vi "ProtocolControl2.vi"() -> ()   [LabVIEW 2016]
uses:
  ProtocolStatus.ctl
  <vilib>/xml/Close Reference(Node).vi
  <vilib>/xml/Load XML File.vi
  <vilib>/xml/NI_XML.lvlib
  <resource>/objmgr/DOMUserDefRef.rc
panel:
  out "Time to Next":dbl format="%#.2f"
  out "Time to Next Subsession":dbl caption="Time to Next"
  out "Current Subsession":string caption="Name"
  out "Time of Current Subsession":dbl caption="Time"
  out "Current Subsession Idx":i32 caption="Index"
  in  "Engage":bool
  in  "Subject ID":string
  out "Pause Time":dbl format="%#.2f"
  out "Record Time":dbl format="%#.2f"
  out "Session Time (s)":dbl
  out "Current Session":dbl(slide) min=0.0 max=600.0 scale=0.0..180.0
  out "Current Time":dbl format="%#.2f"
  out "File Name":string
  out "Suggestions":string
  in  "Close Protocol":bool
  in  "Pause Session":bool
  in  "Start Session":bool
  in  "Load Protocol":bool
  in  "Sessions":i32(listbox)
  in  "XML File Path":path
  # "Current Subsession"
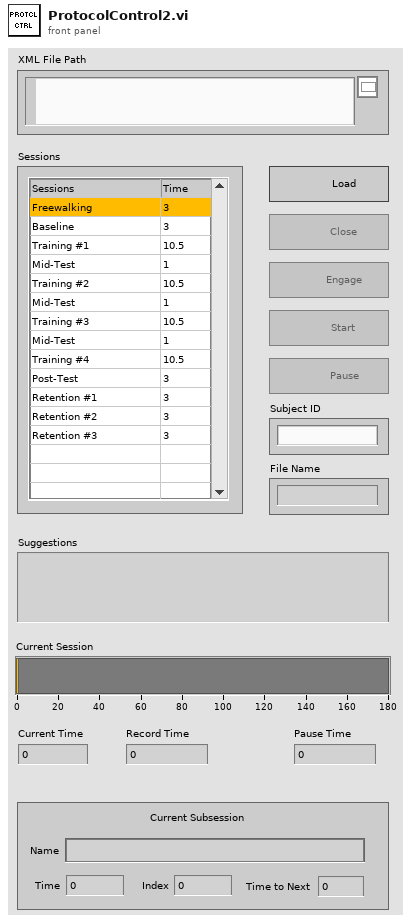
[diagram p1: front panel]
types:
  T1 = typedef "ProtocolStatus.ctl" = enum16{"No Protocol", "Protocol Idle", "Protocol Start", "Protocol Pause"}
  T2 = enum8{"Enabled", "Disabled", "Disabled and Grayed Out"}
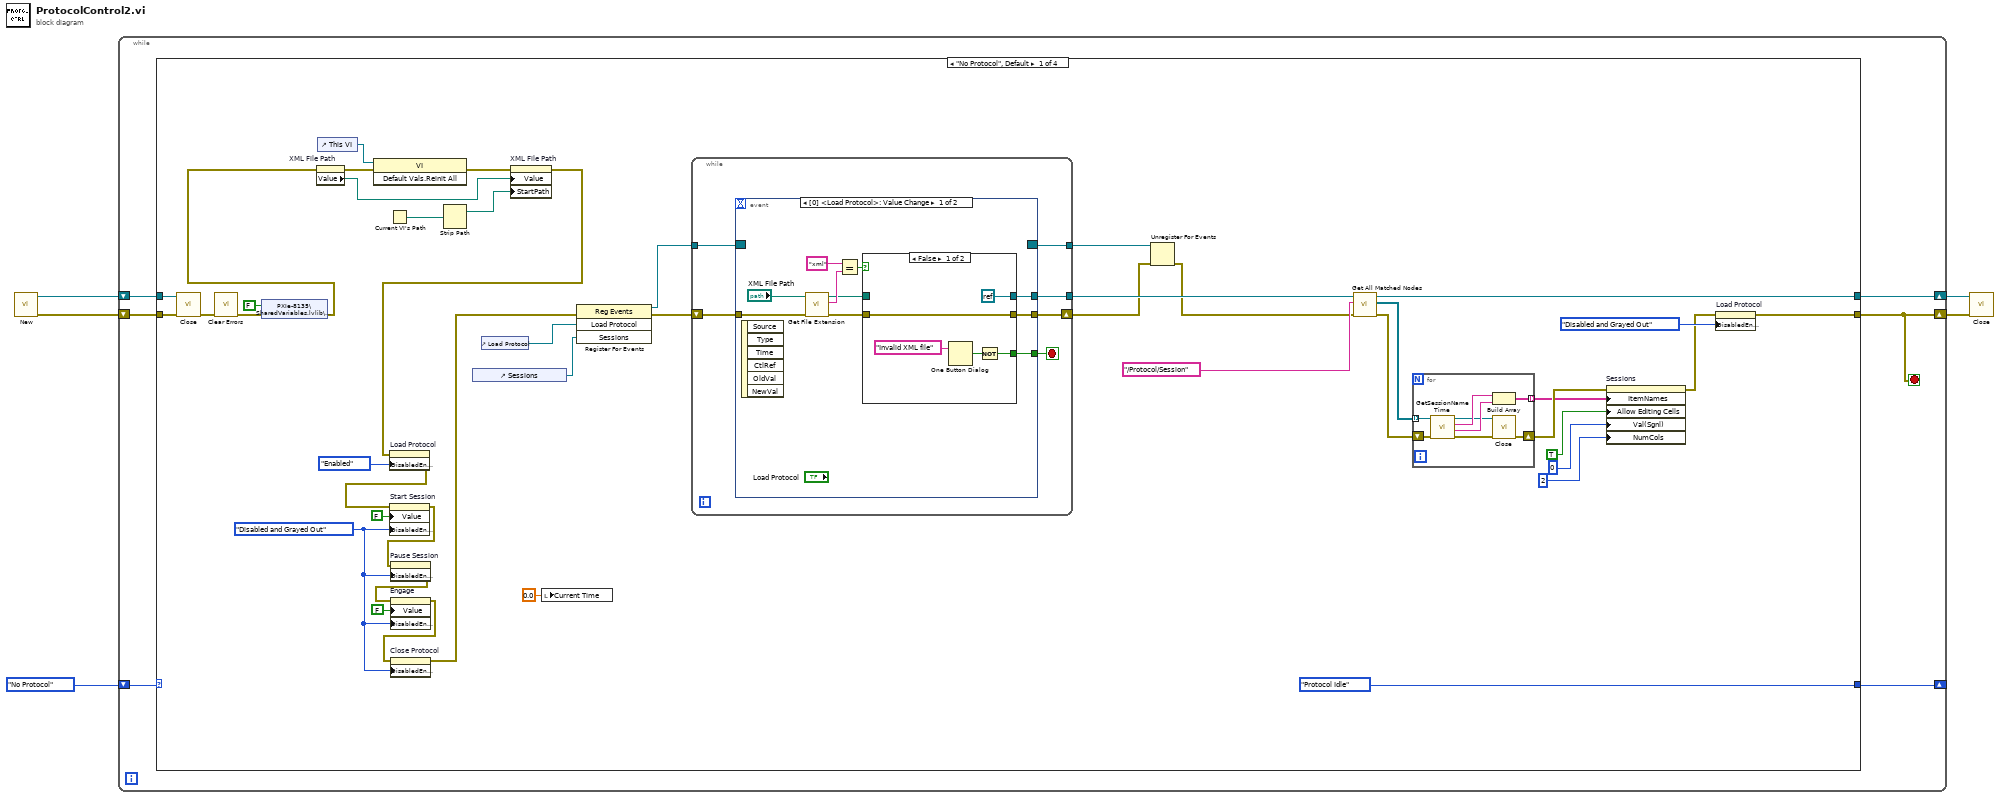
[diagram p0: block diagram]
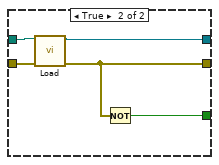
[diagram p2: hidden frame]
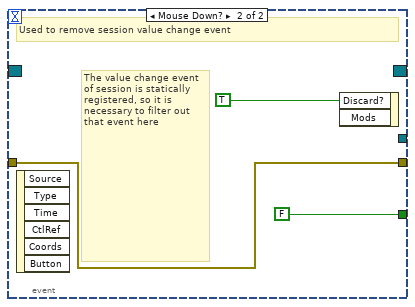
[diagram p3: hidden frame]
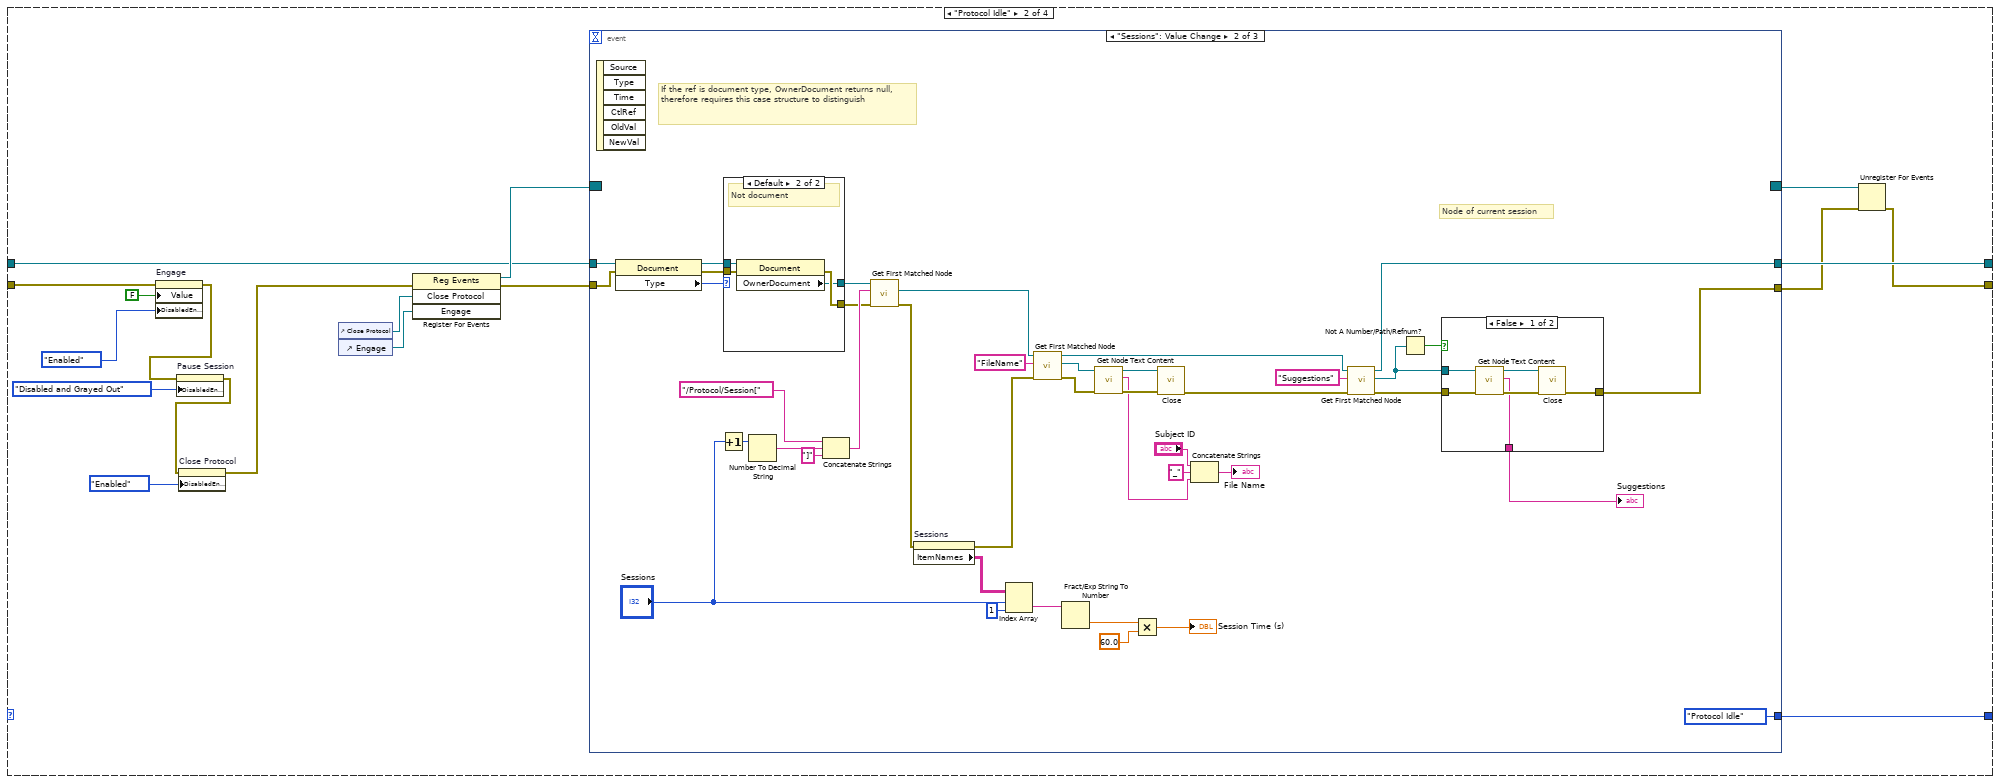
[diagram p4: hidden frame]
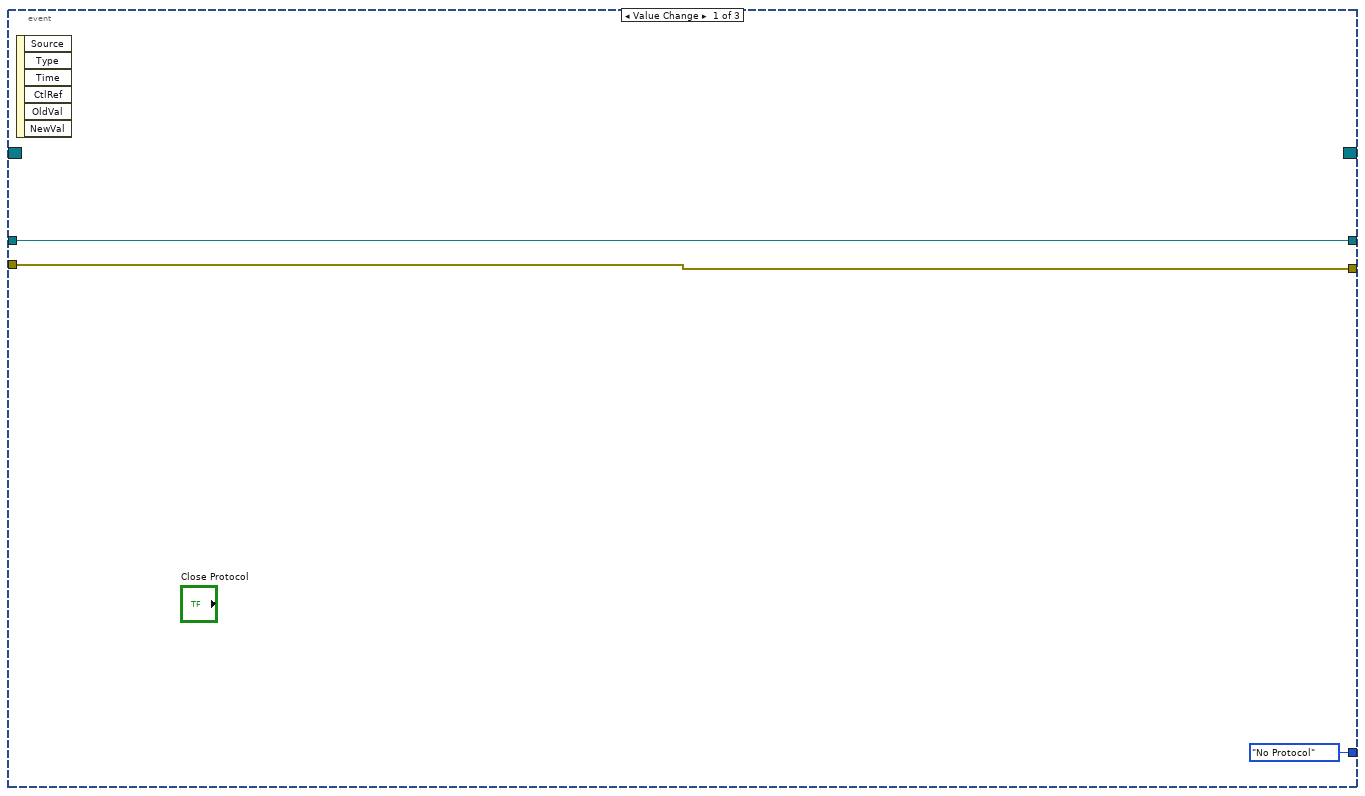
[diagram p5: hidden frame]
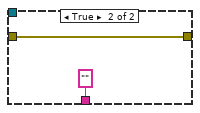
[diagram p7: hidden frame]
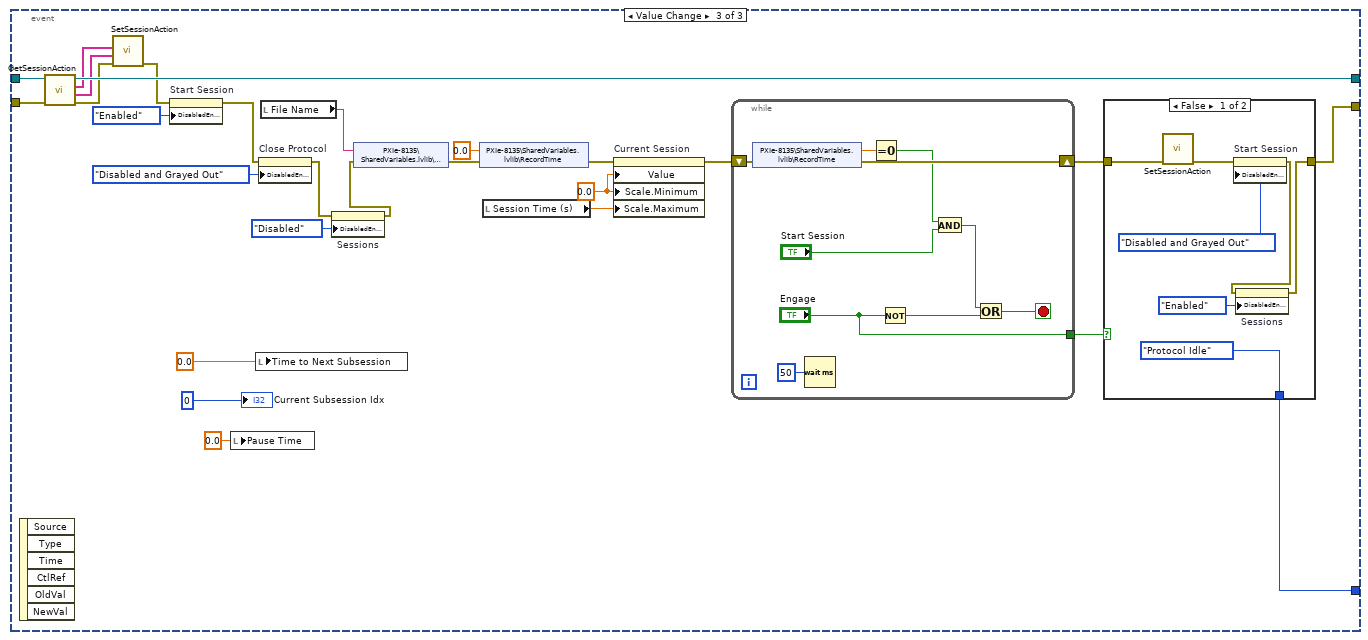
[diagram p8: hidden frame]
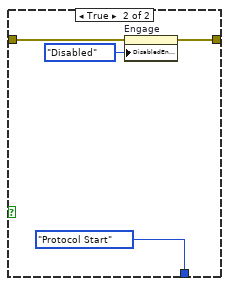
[diagram p9: hidden frame]
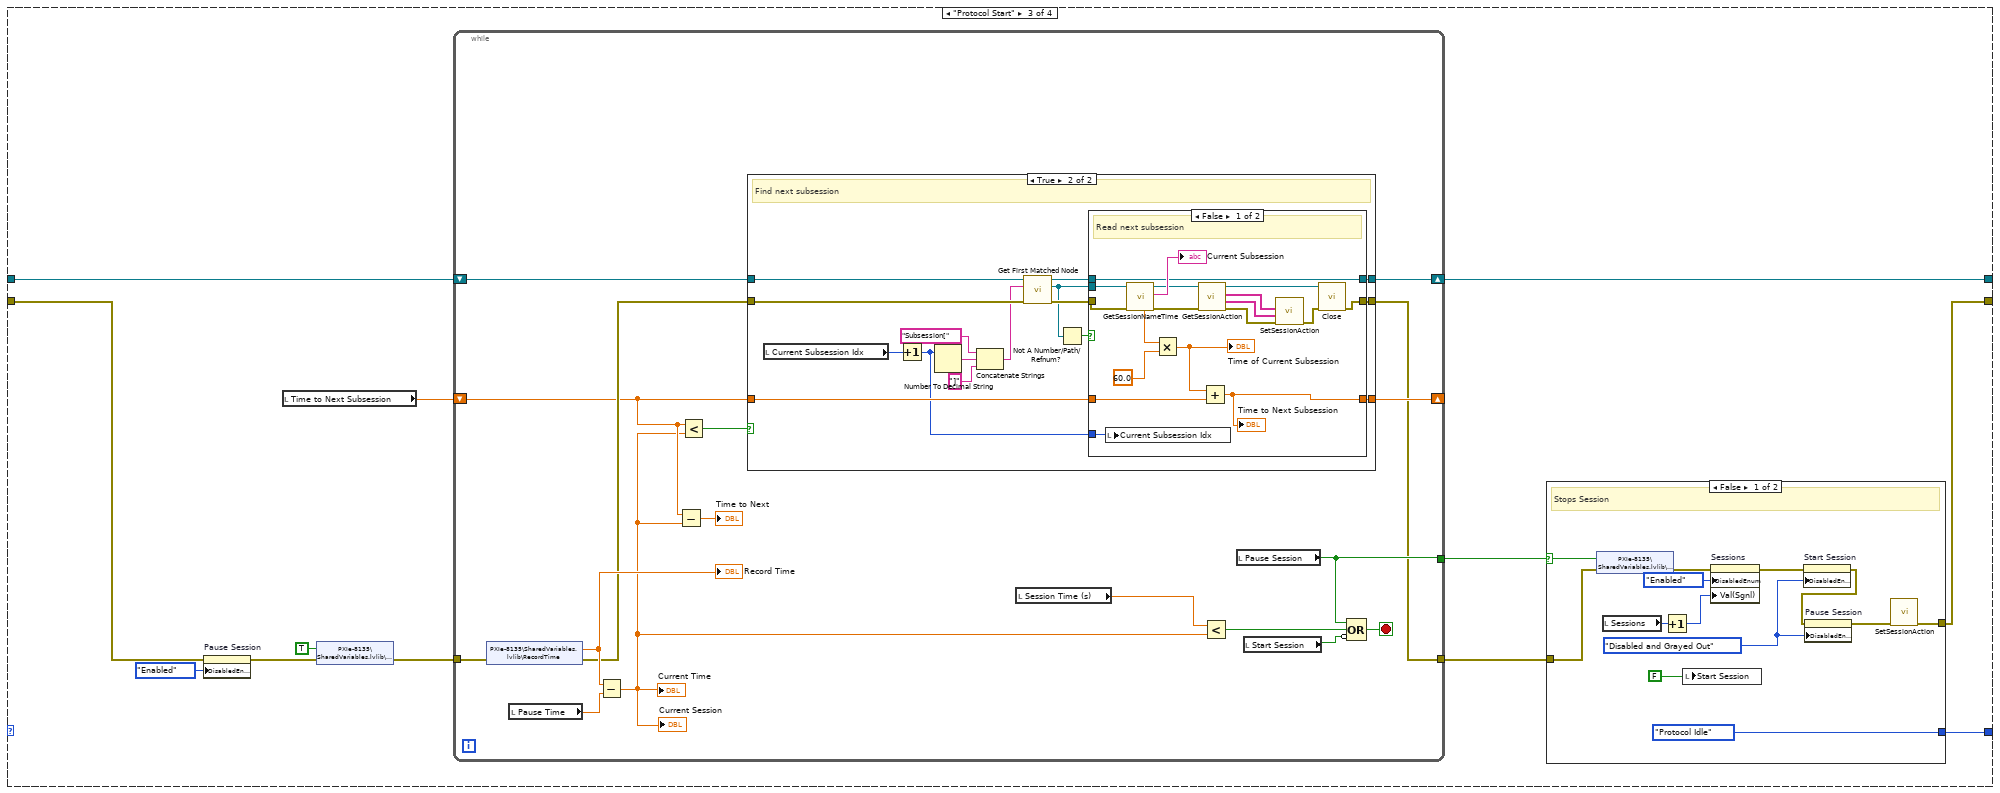
[diagram p10: hidden frame]
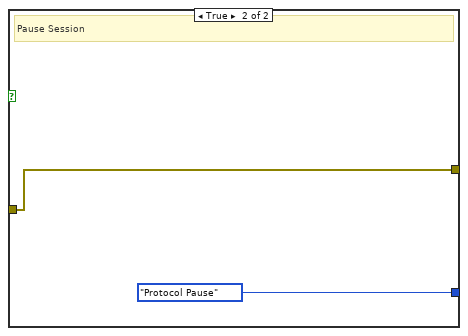
[diagram p11: hidden frame]
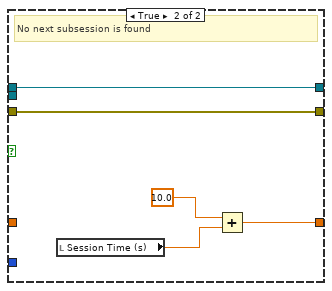
[diagram p13: hidden frame]
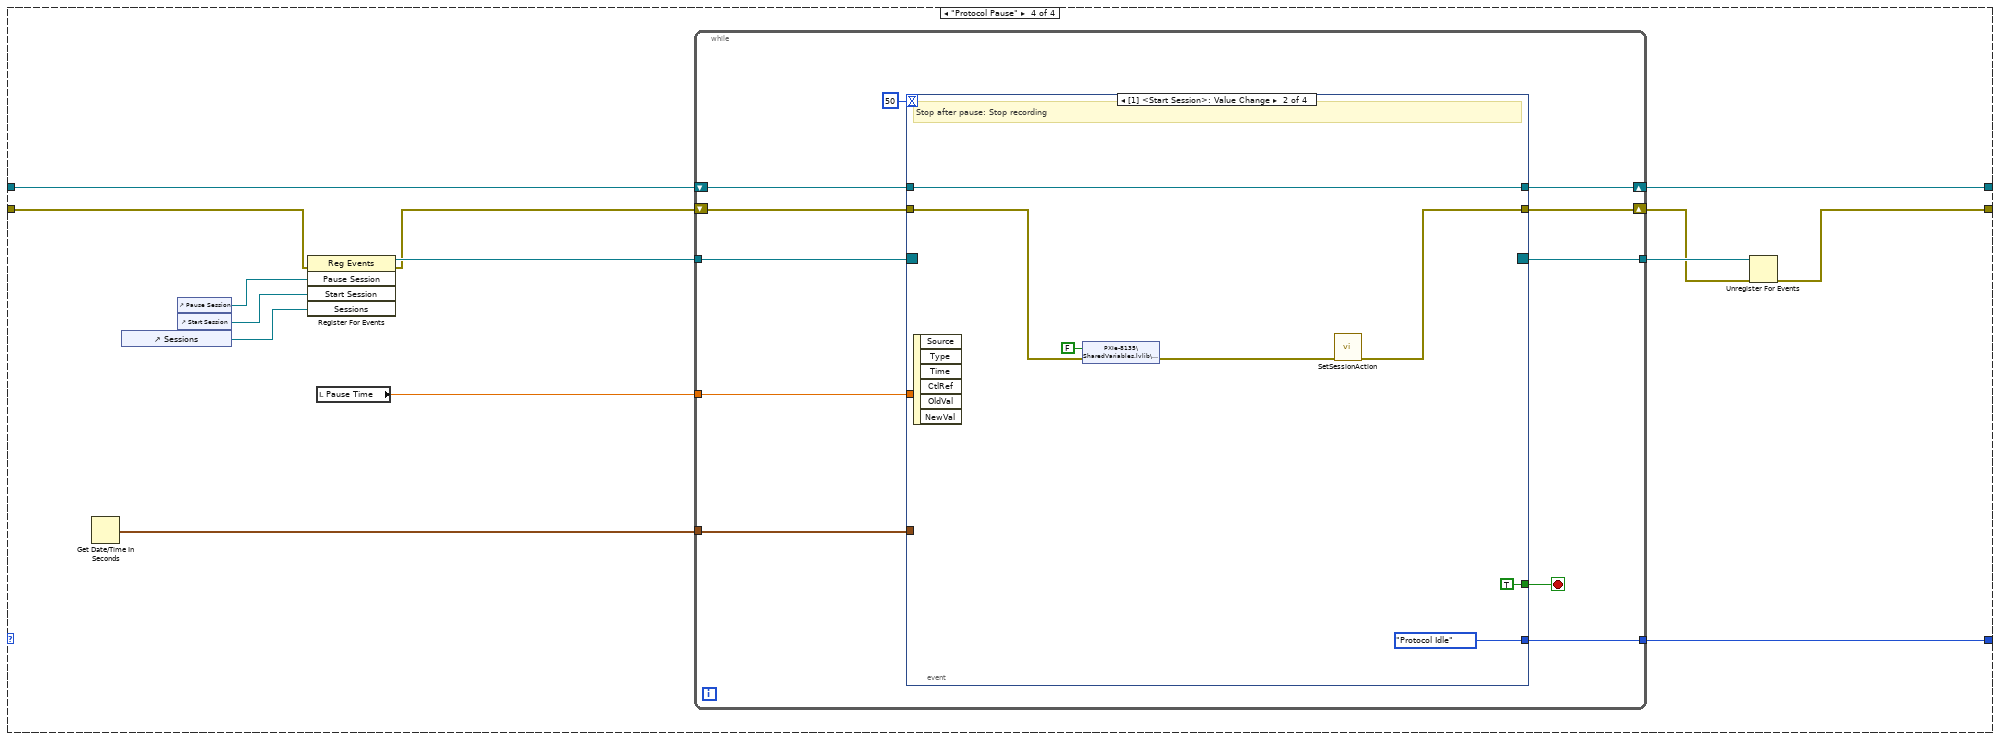
[diagram p14: hidden frame]
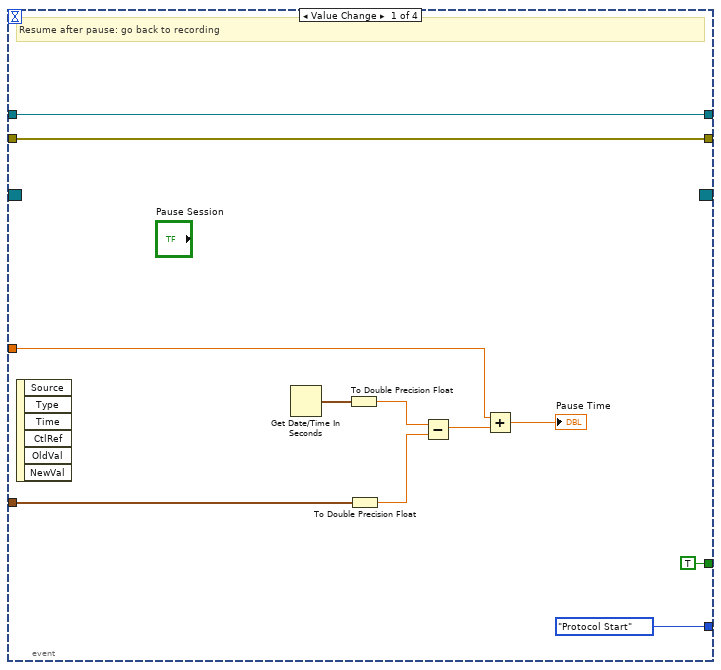
[diagram p15: hidden frame]
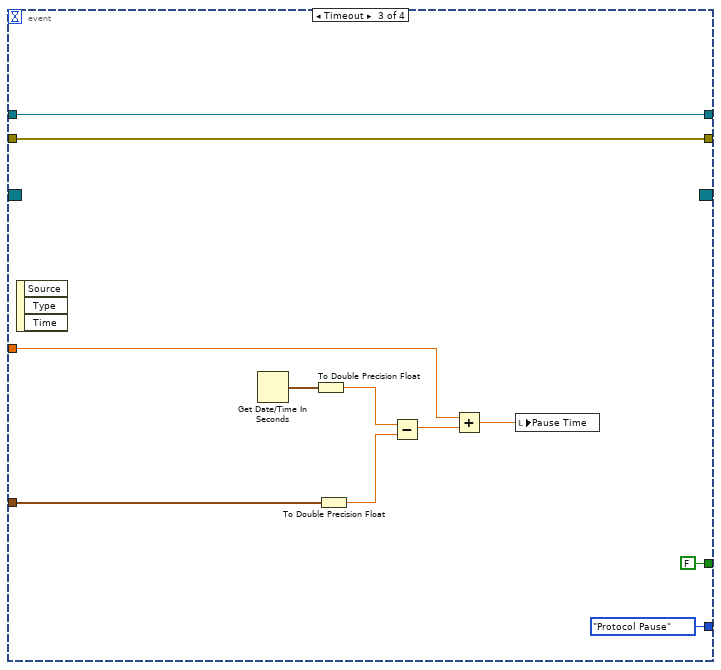
[diagram p16: hidden frame]
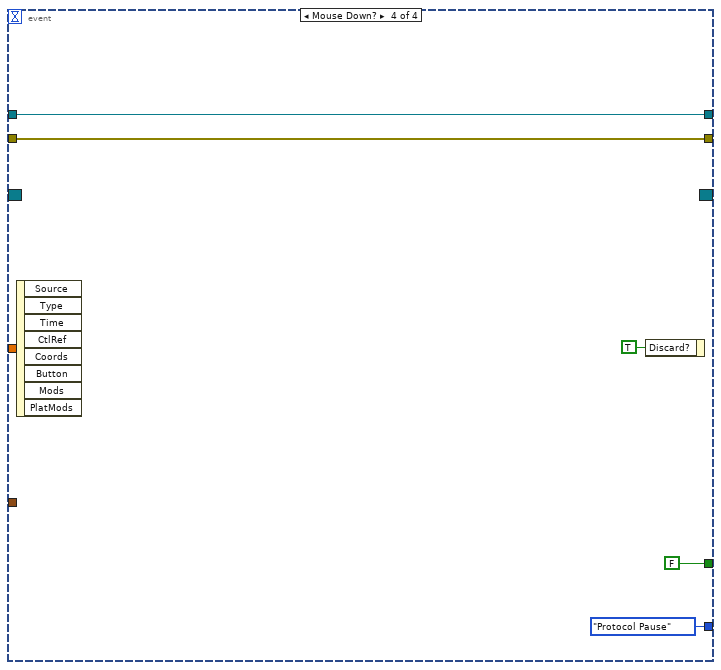
[diagram p17: hidden frame]
diagram:
  n1 = call <vilib>:"New.vi"() -> ("error out"=w3:errorcluster, "DOM document out"=w4:refnum<k20>)  [unwired: 8 in]
  n2 = while {
    shift-right: [w10] -> w2
    shift-left: w4 -> [w9]
    shift-right: [w6] -> w1
    shift-left: w3 -> [w8]
    shift-right: [w7] -> _
    shift-left: ProtocolStatus."No Protocol" -> [w11]
    stop <- w6 stop-if-true
    n3 = case shown="\"No Protocol\", Default" w11 {
      tunnel: [w48 w109 w226 w314] -> w10
      tunnel: w9 -> [w55 w104 w219 w315]
      tunnel: w8 -> [w54 w102 w218 w308]
      tunnel: [w24 w94 w223 w304] -> w6
      tunnel: [ProtocolStatus."Protocol Idle" w110 w222 w316] -> w7
      frame "No Protocol", Default {
        w25 = T2."Disabled and Grayed Out" ("Disabled")
        n4 = call-poly <vilib>:"Close.vi"("error in (no error)"=w54, "node"=w55) -> ("error out"=w21:errorcluster)  [unwired: 7 in]
        n5 = call <vilib>:"Clear Errors.vi"("error in (no error)"=w21) -> ("error out"=w20:errorcluster)  [unwired: 5 in, 1 out]
        n6 = shared-variable "PXIe-8135\\SharedVariables.lvlib\\Record?"(FALSE ("Record?"), error in=w20) -> (error out=w18:errorcluster)
        n7 = property on="XML File Path" class="Path"(error in=w18) -> (error out=w14:errorcluster, "Value"=w13:path)  [unwired: 1 in, 1 out]
        n8 = control-ref of="This VI"() -> (w16:refnum<vi>)
        n9 = invoke class="VI" method="Default Vals.Reinit All"(reference=w16, error in=w14) -> (error out=w15:errorcluster)  [unwired: 1 in, 2 out]
        n10 = Current VI's Path() -> (path=w17:path)
        n11 = Strip Path(path=w17) -> (stripped path=w12:path)  [unwired: 1 out]
        n12 = control-ref of="Sessions"() -> (w36:refnum<vi>)
        n13 = control-ref of="Load Protocol"() -> (w35:refnum<vi>)
        n14 = property on="XML File Path" class="Path"(error in=w15, "Value"=w13, "StartPath"=w12) -> (error out=w19:errorcluster)  [unwired: 1 in, 1 out]
        n15 = property on="Load Protocol" class="Bool"(error in=w19, "DisabledEnum"=T2."Enabled" ("Disabled")) -> (error out=w37:errorcluster)  [unwired: 1 in, 1 out]
        n16 = property on="Start Session" class="Bool (strict)"(error in=w37, "Value"=FALSE ("Start Session"), "DisabledEnum"=w25) -> (error out=w29:errorcluster)  [unwired: 1 in, 1 out]
        n17 = property on="Pause Session" class="Bool (strict)"(error in=w29, "DisabledEnum"=w25) -> (error out=w28:errorcluster)  [unwired: 1 in, 1 out]
        n18 = property on="Engage" class="Bool (strict)"(error in=w28, "Value"=FALSE ("Engage"), "DisabledEnum"=w25) -> (error out=w27:errorcluster)  [unwired: 1 in, 1 out]
        n19 = property on="Close Protocol" class="Bool"(error in=w27, "DisabledEnum"=w25) -> (error out=w26:errorcluster)  [unwired: 1 in, 1 out]
        n20 = local write "Current Time"(0.0 ("Current Time")) -> ()
        n21 = register-events(error in=w26, w35, w36) -> (reference out=w33:refnum<event-registration>, error out=w34:errorcluster)  [unwired: 1 in]
        n22 = while {
          tunnel: [w61] -> w49
          shift-right: [w58] -> w31
          shift-left: w34 -> [w56]
          tunnel: w33 -> [w59]
          tunnel: [w57] -> w32
          stop <- w60 stop-if-true
          n23 = event shown="[0] <Load Protocol>: Value Change" {
            selector: w59 -> [_ _]
            dyn-events: [_ _] -> w57
            timeout: _ -> [_ _]
            tunnel: [w63 _] -> w61
            tunnel: w56 -> [w67 w82]
            tunnel: [w62 FALSE] -> w60
            tunnel: [w64 w82] -> w58
            event Value Change {
              n24 = event-data() -> ()  [unwired: 1 in, 6 out]
              n25 = call <vilib>:"Get File Extension.vi"("error in (no error)"=w67, "file"="XML File Path") -> ("error out"=w66:errorcluster, "lowercase file extension"=w68:string, "dup file"=w65:path)  [unwired: 5 in, 2 out]
              n26 = Equal?(x="xml" ("y"), y=w68) -> (x = y?=w71:bool)
              n27 = case shown="False" w71 {
                tunnel: w66 -> [w75 w80]
                tunnel: w65 -> [_ w81]
                tunnel: [w75 w78] -> w64
                tunnel: [refnum<k0> refnum w79] -> w63
                tunnel: [w73 w77] -> w62
                frame False {
                  n28 = One Button Dialog(message="Invalid XML file") -> (true=w74:bool)  [unwired: 1 in]
                  n29 = Not(x=w74) -> (.not. x?=w73:bool)
                }
                frame True {
                  n30 = call-poly <vilib>:"Load.vi"("path to XML document"=w81, "error in (no error)"=w80) -> ("DOM document out"=w79:refnum<k20>, "error out"=w78:errorcluster)  [unwired: 11 in, 1 out]
                  n31 = Not(x=w78) -> (.not. x?=w77:bool)
                }
              }
            }
            event Mouse Down? {
              # "The value change event of session is statically registered, so it is necessary to filter out that event here"
              # "Used to remove session value change event"
              n32 = event-data() -> ()  [unwired: 1 in, 6 out]
              n33 = event-data("Discard?"=TRUE) -> ()  [unwired: 2 in, 1 out]
            }
          }
        }
        n34 = Unregister For Events(event registration refnum=w32, error in=w31) -> (error out=w30:errorcluster)
        n35 = call <vilib>:"Get All Matched Nodes.vi"("error in (no error)"=w30, "XPath expression"="/Protocol/Session", "node in"=w49) -> ("error out"=w52:errorcluster, "node result array"=w50:refnum<k20>[], "node out"=w48:refnum<k20>)  [unwired: 6 in]
        n36 = for {
          tunnel: w50 -> [w85] mode=indexing
          shift-right: [w86] -> w47
          shift-left: w52 -> [w92]
          tunnel: [w89] -> w43 mode=indexing
          n37 = call "GetSessionNameTime.vi"("error in (no error)"=w92, "Refnum in"=w85) -> ("error out"=w88:errorcluster, "Session Time"=w91:string, "Session Name"=w90:string, "node out"=w87:refnum<k20>)  [unwired: 5 in, 1 out]
          n38 = Build Array(w90, w91) -> (w89:string[])
          n39 = call-poly <vilib>:"Close.vi"("error in (no error)"=w88, "node"=w87) -> ("error out"=w86:errorcluster)  [unwired: 7 in]
        }
        n40 = property on="Sessions" class="MCListbox (strict)"(error in=w47, "ItemNames"=w43, "Allow Editing Cells"=TRUE, "Val(Sgnl)"=0 ("Protocol"), "NumCols"=u32 2 ("Number of Columns")) -> (error out=w39:errorcluster)  [unwired: 1 in, 1 out]
        n41 = property on="Load Protocol" class="Bool"(error in=w39, "DisabledEnum"=T2."Disabled and Grayed Out" ("Disabled")) -> (error out=w24:errorcluster)  [unwired: 1 in, 1 out]
      }
      frame "Protocol Idle" {
        n42 = property on="Engage" class="Bool (strict)"(error in=w102, "Value"=FALSE ("Engage"), "DisabledEnum"=T2."Enabled" ("Disabled")) -> (error out=w99:errorcluster)  [unwired: 1 in, 1 out]
        n43 = property on="Pause Session" class="Bool (strict)"(error in=w99, "DisabledEnum"=T2."Disabled and Grayed Out" ("Disabled")) -> (error out=w96:errorcluster)  [unwired: 1 in, 1 out]
        n44 = property on="Close Protocol" class="Bool"(error in=w96, "DisabledEnum"=T2."Enabled" ("Disabled")) -> (error out=w93:errorcluster)  [unwired: 1 in, 1 out]
        n45 = control-ref of="Close Protocol"() -> (w107:refnum<vi>)
        n46 = control-ref of="Engage"() -> (w103:refnum<vi>)
        n47 = register-events(error in=w93, w107, w103) -> (reference out=w106:refnum<event-registration>, error out=w108:errorcluster)  [unwired: 1 in]
        n48 = event shown="[1] \"Sessions\": Value Change" {
          selector: w106 -> [_ _ _]
          dyn-events: [_ _ _] -> w105
          timeout: _ -> [_ _ _]
          tunnel: [ProtocolStatus."No Protocol" ProtocolStatus."Protocol Idle" w181] -> w110
          tunnel: w104 -> [w113 w127 w178]
          tunnel: w108 -> [w112 w126 w177]
          tunnel: [w112 w129 w183] -> w95
          tunnel: [w113 w128 w176] -> w109
          event Value Change {
            n49 = event-data() -> ()  [unwired: 1 in, 6 out]
          }
          event "Sessions": Value Change {
            # "If the ref is document type, OwnerDocument returns null, therefore requires this case structure to distinguish"
            # "Node of current session"
            n50 = event-data() -> ()  [unwired: 1 in, 6 out]
            n51 = property class="Document"(reference=w127, error in=w126) -> (reference out=w122:refnum<k20>, error out=w124:errorcluster, "Type"=w125:i32)
            n52 = Increment(x="Sessions") -> (x+1=w133:i32)
            n53 = case shown="Default" w125 {
              tunnel: [w156 w158] -> w123
              tunnel: w124 -> [w156 w159]
              tunnel: w122 -> [w155 w160]
              tunnel: [w155 w157] -> w121
              frame 9 {
                # "Document Type"
              }
              frame Default {
                # "Not document"
                n54 = property class="Document"(reference=w160, error in=w159) -> (error out=w158:errorcluster, "OwnerDocument"=w157:refnum<k20>)  [unwired: 1 out]
              }
            }
            n55 = Number To Decimal String(number=w133) -> (decimal integer string=w136:string)  [unwired: 1 in]
            n56 = Concatenate Strings("/Protocol/Session[" ("XPath expression"), w136, "]" ("string")) -> (w135:string)
            n57 = call <vilib>:"Get First Matched Node.vi"("error in (no error)"=w123, "XPath expression"=w135, "node in"=w121) -> ("error out"=w131:errorcluster, "node result"=w130:refnum<k20>)  [unwired: 6 in, 1 out]
            n58 = property on="Sessions" class="MCListbox (strict)"(error in=w131) -> (error out=w137:errorcluster, "ItemNames"=w142:string[][])  [unwired: 1 in, 1 out]
            n59 = Index Array(array=w142, index (row)="Sessions", index (col)=1 ("disabled index (col)")) -> (element=w140:string)
            n60 = call <vilib>:"Get First Matched Node.vi"("error in (no error)"=w137, "XPath expression"="FileName", "node in"=w130) -> ("error out"=w152:errorcluster, "node result"=w153:refnum<k20>, "node out"=w143:refnum<k20>)  [unwired: 6 in]
            n61 = Fract/Exp String To Number(string=w140) -> (number=w139:dbl)  [unwired: 3 in, 1 out]
            n62 = call <vilib>:"Get Node Text Content.vi"("error in (no error)"=w152, "node in"=w153) -> ("error out"=w151:errorcluster, "node text"=w117:string, "node out"=w150:refnum<k20>)  [unwired: 7 in]
            n63 = Multiply(x=w139, y=60.0) -> (x*y=→"Session Time (s)":dbl)
            n64 = call-poly <vilib>:"Close.vi"("error in (no error)"=w151, "node"=w150) -> ("error out"=w138:errorcluster)  [unwired: 7 in]
            n65 = Concatenate Strings("Subject ID", "_" ("string"), w117) -> (→"File Name":string)
            n66 = call <vilib>:"Get First Matched Node.vi"("error in (no error)"=w138, "XPath expression"="Suggestions", "node in"=w143) -> ("error out"=w148:errorcluster, "node result"=w146:refnum<k20>, "node out"=w128:refnum<k20>)  [unwired: 6 in]
            n67 = Not A Number/Path/Refnum?(number/path/refnum=w146) -> (NaN/Path/Refnum?=w145:bool)
            n68 = case shown="False" w145 {
              tunnel: w148 -> [w164 w168]
              tunnel: w146 -> [w163 _]
              tunnel: [w162 "" ("node text")] -> w144
              tunnel: [w161 w168] -> w129
              frame False {
                n69 = call <vilib>:"Get Node Text Content.vi"("error in (no error)"=w164, "node in"=w163) -> ("error out"=w165:errorcluster, "node text"=w162:string, "node out"=w166:refnum<k20>)  [unwired: 7 in]
                n70 = call-poly <vilib>:"Close.vi"("error in (no error)"=w165, "node"=w166) -> ("error out"=w161:errorcluster)  [unwired: 7 in]
              }
              frame True {
              }
            }
            "Suggestions" <- w144
          }
          event Value Change {
            w194 = 0.0 ("Data Entry Limits:Minimum")
            n71 = event-data() -> ()  [unwired: 1 in, 6 out]
            n72 = call "GetSessionAction.vi"("error in (no error)"=w177, "Refnum in"=w178) -> ("error out"=w173:errorcluster, "ActionValue"=w174:string[], "ActionName"=w175:string[], "node out"=w176:refnum<k20>)  [unwired: 6 in]
            n73 = call "SetSessionAction.vi"("error in (no error)"=w173, "ActionValue (False)"=w174, "ActionName  (ForceField)"=w175) -> ("error out"=w172:errorcluster)  [unwired: 8 in]
            n74 = property on="Start Session" class="Bool (strict)"(error in=w172, "DisabledEnum"=T2."Enabled" ("Disabled")) -> (error out=w185:errorcluster)  [unwired: 1 in, 1 out]
            n75 = local write "Pause Time"(0.0 ("Pause Time")) -> ()
            n76 = local write "Time to Next Subsession"(0.0 ("Time to Start Next Subsession")) -> ()
            n77 = property on="Close Protocol" class="Bool"(error in=w185, "DisabledEnum"=T2."Disabled and Grayed Out" ("Disabled")) -> (error out=w171:errorcluster)  [unwired: 1 in, 1 out]
            n78 = local read "File Name"() -> (w189:string)
            n79 = property on="Sessions" class="MCListbox (strict)"(error in=w171, "DisabledEnum"=T2."Disabled" ("Disabled")) -> (error out=w170:errorcluster)  [unwired: 1 in, 1 out]
            n80 = shared-variable "PXIe-8135\\SharedVariables.lvlib\\FileName"(w189, error in=w170) -> (error out=w190:errorcluster)
            n81 = shared-variable "PXIe-8135\\SharedVariables.lvlib\\RecordTime"(0.0 ("RecordTime"), error in=w190) -> (error out=w180:errorcluster)
            n82 = local read "Session Time (s)"() -> (w192:dbl)
            n83 = property on="Current Session" class="Slide (strict)"(error in=w180, "Value"=w194, "Scale.Minimum"=w194, "Scale.Maximum"=w192) -> (error out=w179:errorcluster)  [unwired: 1 in, 1 out]
            n84 = while {
              tunnel: ["Engage"] -> w182
              shift-right: [w215] -> w184
              shift-left: w179 -> [w216]
              stop <- w207 stop-if-true
              n85 = shared-variable "PXIe-8135\\SharedVariables.lvlib\\RecordTime"(error in=w216) -> (w214:dbl, error out=w215:errorcluster)
              n86 = Wait (ms)(milliseconds to wait=u32 50) -> ()  [unwired: 1 out]
              n87 = Equal To 0?(x=w214) -> (x = 0?=w212:bool)
              n88 = Not(x="Engage") -> (.not. x?=w210:bool)
              n89 = And(x=w212, y="Start Session") -> (x .and. y?=w211:bool)
              n90 = Or(x=w211, y=w210) -> (x .or. y?=w207:bool)
            }
            n91 = case shown="False" w182 {
              tunnel: w184 -> [w200 w205]
              tunnel: [w196 w204] -> w183
              tunnel: [ProtocolStatus."Protocol Idle" ProtocolStatus."Protocol Start"] -> w181
              frame False {
                n92 = call "SetSessionAction.vi"("error in (no error)"=w200) -> ("error out"=w199:errorcluster)  [unwired: 10 in]
                n93 = property on="Start Session" class="Bool (strict)"(error in=w199, "DisabledEnum"=T2."Disabled and Grayed Out" ("Disabled")) -> (error out=w197:errorcluster)  [unwired: 1 in, 1 out]
                n94 = property on="Sessions" class="MCListbox (strict)"(error in=w197, "DisabledEnum"=T2."Enabled" ("Disabled")) -> (error out=w196:errorcluster)  [unwired: 1 in, 1 out]
              }
              frame True {
                n95 = property on="Engage" class="Bool (strict)"(error in=w205, "DisabledEnum"=T2."Disabled" ("Disabled")) -> (error out=w204:errorcluster)  [unwired: 1 in, 1 out]
              }
            }
            "Current Subsession Idx" <- 0 ("Current Subsession Idx")
          }
        }
        n96 = Unregister For Events(event registration refnum=w105, error in=w95) -> (error out=w94:errorcluster)
      }
      frame "Protocol Start" {
        n97 = property on="Pause Session" class="Bool (strict)"(error in=w218, "DisabledEnum"=T2."Enabled" ("Disabled")) -> (error out=w221:errorcluster)  [unwired: 1 in, 1 out]
        n98 = local read "Time to Next Subsession"() -> (w217:dbl)
        n99 = shared-variable "PXIe-8135\\SharedVariables.lvlib\\Record?"(TRUE ("Record?"), error in=w221) -> (error out=w228:errorcluster)
        n100 = while {
          tunnel: w228 -> [w260]
          shift-right: [w257] -> _
          shift-left: w217 -> [w246]
          tunnel: [w247] -> w224
          tunnel: [w251] -> w225
          shift-right: [w258] -> w226
          shift-left: w219 -> [w254]
          stop <- w252 stop-if-true
          n101 = shared-variable "PXIe-8135\\SharedVariables.lvlib\\RecordTime"(error in=w260) -> (w256:dbl, error out=w248:errorcluster)
          "Record Time" <- w256
          n102 = local read "Pause Time"() -> (w259:dbl)
          n103 = Subtract(x=w256, y=w259) -> (x-y=w245:dbl)
          "Current Session" <- w245
          "Current Time" <- w245
          n104 = Subtract(x=w246, y=w245) -> (x-y=→"Time to Next":dbl)
          n105 = Less?(x=w246, y=w245) -> (x < y?=w253:bool)
          n106 = case shown="True" w253 {
            tunnel: w254 -> [w262 w277]
            tunnel: [w262 w276] -> w258
            tunnel: w246 -> [w263 w279]
            tunnel: [w263 w278] -> w257
            tunnel: w248 -> [w261 w274]
            tunnel: [w261 w273] -> w247
            frame False {
            }
            frame True {
              # "Find next subsession"
              n107 = local read "Current Subsession Idx"() -> (w269:i32)
              n108 = Increment(x=w269) -> (x+1=w264:i32)
              n109 = Number To Decimal String(number=w264) -> (decimal integer string=w268:string)  [unwired: 1 in]
              n110 = Concatenate Strings("Subsession[", w268, "]") -> (w265:string)
              n111 = call <vilib>:"Get First Matched Node.vi"("error in (no error)"=w274, "XPath expression"=w265, "node in"=w277) -> ("error out"=w275:errorcluster, "node result"=w270:refnum<k20>, "node out"=w272:refnum<k20>)  [unwired: 6 in]
              n112 = Not A Number/Path/Refnum?(number/path/refnum=w270) -> (NaN/Path/Refnum?=w271:bool)
              n113 = case shown="False" w271 {
                tunnel: w279 -> [w295 _]
                tunnel: [w280 w301] -> w278
                tunnel: w270 -> [w294 _]
                tunnel: [w290 w298] -> w276
                tunnel: w275 -> [w293 w299]
                tunnel: [w289 w299] -> w273
                tunnel: w272 -> [w290 w298]
                tunnel: w264 -> [w288 _]
                frame False {
                  # "Read next subsession"
                  n114 = local write "Current Subsession Idx"(w288) -> ()
                  n115 = call "GetSessionNameTime.vi"("error in (no error)"=w293, "Refnum in"=w294) -> ("error out"=w283:errorcluster, "Session Name"=→"Current Subsession":string, "node out"=w284:refnum<k20>, "Session Time (min)"=w296:dbl)  [unwired: 5 in, 1 out]
                  n116 = Multiply(x=w296, y=60.0) -> (x*y=w292:dbl)
                  "Time of Current Subsession" <- w292
                  n117 = call "GetSessionAction.vi"("error in (no error)"=w283, "Refnum in"=w284) -> ("error out"=w285:errorcluster, "ActionValue"=w286:string[], "ActionName"=w287:string[], "node out"=w281:refnum<k20>)  [unwired: 6 in]
                  n118 = Add(x=w292, y=w295) -> (x+y=w280:dbl)
                  "Time to Next Subsession" <- w280
                  n119 = call "SetSessionAction.vi"("error in (no error)"=w285, "ActionValue (False)"=w286, "ActionName  (ForceField)"=w287) -> ("error out"=w282:errorcluster)  [unwired: 8 in]
                  n120 = call-poly <vilib>:"Close.vi"("error in (no error)"=w282, "node"=w281) -> ("error out"=w289:errorcluster)  [unwired: 7 in]
                }
                frame True {
                  # "No next subsession is found"
                  n121 = local read "Session Time (s)"() -> (w302:dbl)
                  n122 = Add(x=10.0, y=w302) -> (x+y=w301:dbl)
                }
              }
            }
          }
          n123 = local read "Session Time (s)"() -> (w255:dbl)
          n124 = Less?(x=w255, y=w245) -> (x < y?=w250:bool)
          n125 = local read "Pause Session"() -> (w251:bool)
          n126 = local read "Start Session"() -> (w249:bool)
          n127 = Compound Arithmetic op=OR(w251, w250, invert w249) -> (w252:bool)
        }
        n128 = case shown="False" w225 {
          selector: w225 -> [w241 _]
          tunnel: w224 -> [w240 w242]
          tunnel: [w231 w242] -> w223
          tunnel: [ProtocolStatus."Protocol Idle" ProtocolStatus."Protocol Pause"] -> w222
          frame False {
            w234 = T2."Disabled and Grayed Out" ("Disabled")
            # "Stops Session"
            n129 = shared-variable "PXIe-8135\\SharedVariables.lvlib\\Record?"(w241, error in=w240) -> (error out=w237:errorcluster)
            n130 = local read "Sessions"() -> (w238:i32)
            n131 = Increment(x=w238) -> (x+1=w230:i32)
            n132 = local write "Start Session"(FALSE ("Start Session 2")) -> ()
            n133 = property on="Sessions" class="MCListbox (strict)"(error in=w237, "DisabledEnum"=T2."Enabled" ("Disabled"), "Val(Sgnl)"=w230) -> (error out=w235:errorcluster)  [unwired: 1 in, 1 out]
            n134 = property on="Start Session" class="Bool (strict)"(error in=w235, "DisabledEnum"=w234) -> (error out=w233:errorcluster)  [unwired: 1 in, 1 out]
            n135 = property on="Pause Session" class="Bool (strict)"(error in=w233, "DisabledEnum"=w234) -> (error out=w232:errorcluster)  [unwired: 1 in, 1 out]
            n136 = call "SetSessionAction.vi"("error in (no error)"=w232) -> ("error out"=w231:errorcluster)  [unwired: 10 in]
          }
          frame True {
            # "Pause Session"
          }
        }
      }
      frame "Protocol Pause" {
        n137 = Get Date/Time In Seconds() -> (seconds since 1Jan1904=w313:timestamp)
        n138 = control-ref of="Sessions"() -> (w312:refnum<vi>)
        n139 = control-ref of="Pause Session"() -> (w310:refnum<vi>)
        n140 = control-ref of="Start Session"() -> (w311:refnum<vi>)
        n141 = register-events(error in=w308, w310, w311, w312) -> (reference out=w309:refnum<event-registration>, error out=w307:errorcluster)  [unwired: 1 in]
        n142 = local read "Pause Time"() -> (w303:dbl)
        n143 = while {
          tunnel: [w327] -> w316
          shift-right: [w325] -> w314
          shift-left: w315 -> [w326]
          shift-right: [w318] -> w305
          shift-left: w307 -> [w320]
          tunnel: w313 -> [w322]
          tunnel: w309 -> [w321]
          tunnel: [w319] -> w306
          tunnel: w303 -> [w317]
          stop <- w324 stop-if-true
          n144 = event shown="[1] <Start Session>: Value Change" {
            selector: w321 -> [_ _ _ _]
            dyn-events: [_ _ _ _] -> w319
            timeout: 50 -> [_ _ _ _]
            tunnel: [ProtocolStatus."Protocol Start" ProtocolStatus."Protocol Idle" ProtocolStatus."Protocol Pause" ProtocolStatus."Protocol Pause"] -> w327
            tunnel: w320 -> [w336 w343 w353 w359]
            tunnel: w326 -> [w337 w344 w354 w360]
            tunnel: [w337 w344 w354 w360] -> w325
            tunnel: [w336 w339 w353 w359] -> w318
            tunnel: w322 -> [w334 _ w348 _]
            tunnel: [TRUE ("Discard?") TRUE ("Discard?") FALSE ("Discard?") FALSE ("Discard?")] -> w324
            tunnel: w317 -> [w328 _ w346 _]
            event Value Change {
              # "Resume after pause: go back to recording"
              n145 = event-data() -> ()  [unwired: 1 in, 6 out]
              n146 = Get Date/Time In Seconds() -> (seconds since 1Jan1904=w335:timestamp)
              n147 = To Double Precision Float(number=w335) -> (double precision float=w332:dbl)
              n148 = To Double Precision Float(number=w334) -> (double precision float=w333:dbl)
              n149 = Subtract(x=w332, y=w333) -> (x-y=w331:dbl)
              n150 = Add(x=w328, y=w331) -> (x+y=→"Pause Time":dbl)
            }
            event Value Change {
              # "Stop after pause: Stop recording"
              n151 = event-data() -> ()  [unwired: 1 in, 6 out]
              n152 = shared-variable "PXIe-8135\\SharedVariables.lvlib\\Record?"(FALSE ("Record?"), error in=w343) -> (error out=w340:errorcluster)
              n153 = call "SetSessionAction.vi"("error in (no error)"=w340) -> ("error out"=w339:errorcluster)  [unwired: 10 in]
            }
            event Timeout {
              n154 = event-data() -> ()  [unwired: 1 in, 3 out]
              n155 = Get Date/Time In Seconds() -> (seconds since 1Jan1904=w352:timestamp)
              n156 = To Double Precision Float(number=w352) -> (double precision float=w350:dbl)
              n157 = To Double Precision Float(number=w348) -> (double precision float=w351:dbl)
              n158 = Subtract(x=w350, y=w351) -> (x-y=w349:dbl)
              n159 = Add(x=w346, y=w349) -> (x+y=w347:dbl)
              n160 = local write "Pause Time"(w347) -> ()
            }
            event Mouse Down? {
              n161 = event-data() -> ()  [unwired: 1 in, 8 out]
              n162 = event-data("Discard?"=TRUE) -> ()  [unwired: 1 in, 1 out]
            }
          }
        }
        n163 = Unregister For Events(event registration refnum=w306, error in=w305) -> (error out=w304:errorcluster)
      }
    }
  }
  n164 = call-poly <vilib>:"Close.vi"("error in (no error)"=w1, "node"=w2) -> ()  [unwired: 7 in, 1 out]
